vi "Create_AO_WF.vi"(8 "error in":errorcluster) -> (0 "error out":errorcluster)   [LabVIEW 2025]
panel:
  out "Illumination analog waveforms":waveform(dbl)[](graph) caption="Output Waveform"
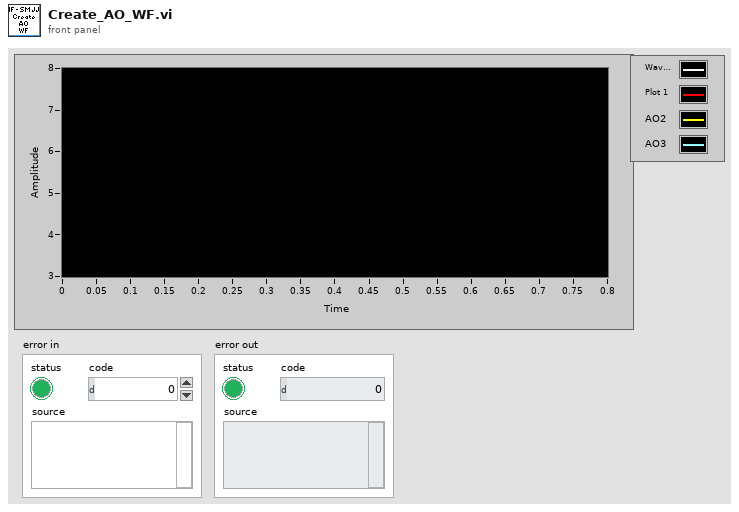
[diagram p1: front panel]
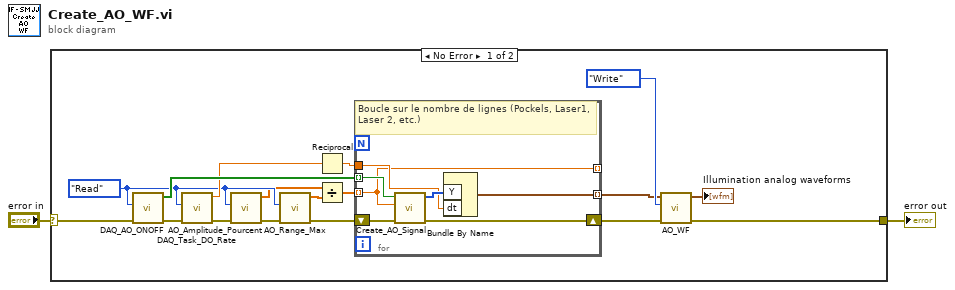
[diagram p0: block diagram]
diagram:
  n1 = case shown="No Error" "error in" {
    selector: "error in" -> [w19 w27]
    tunnel: [w17 w27] -> w1
    frame No Error {
      w7 = enum16{"Write", "Read"}."Read" ("Action")
      n2 = call "DAQ_AO_ONOFF.vi"("error in"=w19, "Action"=w7) -> ("error out"=w13:errorcluster, "AO | ON/OFF"=w15:bool[])  [unwired: 8 in]
      n3 = call "DAQ_Task_DO_Rate.vi"("error in"=w13, "Action"=w7) -> ("error out"=w9:errorcluster, "DO_Rate"=w12:dbl)  [unwired: 8 in]
      n4 = call "AO_Amplitude_Pourcent.vi"("error in"=w9, "Action"=w7) -> ("error out"=w8:errorcluster, "AO | %"=w5:dbl[])  [unwired: 8 in]
      n5 = call "AO_Range_Max.vi"("error in"=w8, "Action"=w7) -> ("error out"=w3:errorcluster, "AO | Max"=w6:dbl[])  [unwired: 8 in]
      n6 = Reciprocal(x=w12) -> (1/x=w10:dbl)
      n7 = Divide(x=w5, y=w6) -> (x/y=w4:dbl[])
      n8 = for {
        shift-right: [w21] -> w18
        shift-left: w3 -> [w26]
        tunnel: w15 -> [w25] mode=indexing
        tunnel: w10 -> [w23]
        tunnel: [w22] -> w11 mode=indexing
        tunnel: [w20] -> _ mode=indexing
        tunnel: w4 -> [w20] mode=indexing
        # "Boucle sur le nombre de lignes (Pockels, Laser1, Laser 2, etc.)"
        n9 = call "Create_AO_Signal.vi"("error in"=w26, "AO Amplitude"=w20, "ON / OFF"=w25) -> ("error out"=w21:errorcluster, "WF"=w24:u32[])  [unwired: 7 in]
        n10 = Bundle By Name("Y"=w24, "dt"=w23) -> (w22:waveform(u32))  [unwired: 1 in]
      }
      n11 = call "AO_WF.vi"("error in"=w18, "Action"=enum16{"Write", "Read"}."Write", "AO WF"=w11) -> ("error out"=w17:errorcluster, "AO WF"=→"Illumination analog waveforms":waveform(dbl)[])  [unwired: 7 in]
    }
    frame Error {
    }
  }
  "error out" <- w1
